vi "NI VeriStand - Close Model.vi"(8 "error in (no error)":errorcluster, 11 "Model":T1) -> (0 "error out":errorcluster)   [LabVIEW 2020, in "NI_VS Model ExecutionAPI.lvlib"]
doc: "Closes an open reference to a model. Use this VI to close each model reference that you open with the Open Model VI."
uses:
  <vilib>/NI VeriStand/Execution/Model/NI_VS Model ExecutionAPI.lvlib
  <vilib>/NI VeriStand/Execution/Model/ModelAPI.ctl
  NationalInstruments.VeriStand.ClientAPI
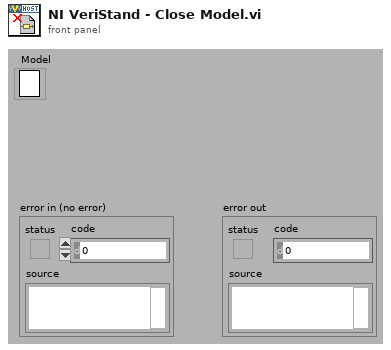
[diagram p1: front panel]
types:
  T1 = typedef "NI_VS Model ExecutionAPI.lvlib/ModelAPI.ctl" = refnum<k24>
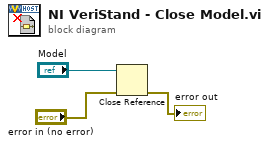
[diagram p0: block diagram]
diagram:
  n1 = Close Reference(reference="Model", error in (no error)="error in (no error)") -> (error out=→"error out":errorcluster)
